vi "Write to TDMS(SubVI).vi"(8 "error in (no error)":errorcluster, 9 "LED state":string, 10 "element":T1 {"RMS" format="%0.6f"; "RPM" format="%0.2f"; "Voltage" format="%0.2f"; "Current" format="%0.2f"; "Temperature" format="%0.2f"}, 11 "Refnum in":refnum<k34>) -> (0 "error out":errorcluster, 3 "Refnum out":refnum<k34>)   [LabVIEW 2017]
uses:
  typedefs/Data.ctl
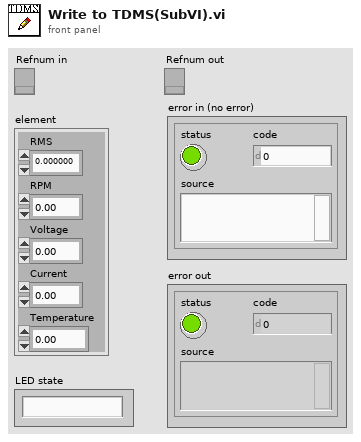
[diagram p1: front panel]
types:
  T1 = typedef "Data.ctl" = cluster{"RMS":dbl, "RPM":dbl, "Voltage":dbl, "Current":dbl, "Temperature":dbl}
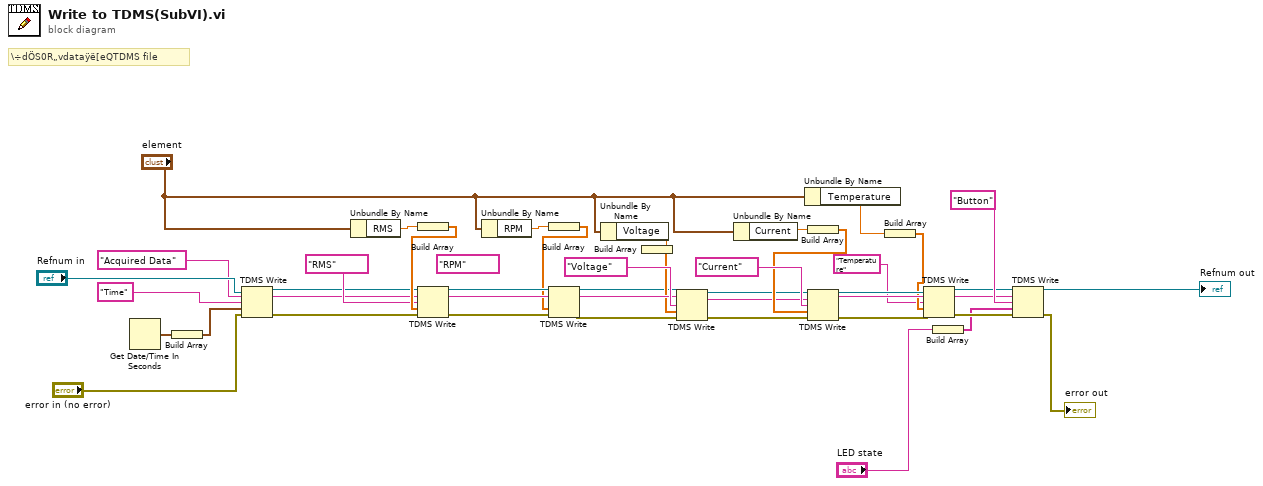
[diagram p0: block diagram]
diagram:
  (unwired) "RPM" ("group name in (Untitled)")
  # "\\÷dÖS0R„vdataÿë[eQTDMS file"
  n1 = Get Date/Time In Seconds() -> (seconds since 1Jan1904=w3:timestamp)
  n2 = Build Array(w3) -> (w4:timestamp[])
  n3 = TDMS Write(0:"Refnum in", 5:"Acquired Data" ("group name in (Untitled)"), 7:"Time" ("group name in (Untitled)"), 9:w4, 11:"error in (no error)") -> (4:w8:refnum<k34>, 6:w6:string, 15:w7:errorcluster)  [unwired: 1 in, 1 out]
  n4 = Unbundle By Name("element") -> ("RMS"=w9:dbl)
  n5 = Build Array(w9) -> (w11:dbl[])
  n6 = TDMS Write(0:w8, 5:w6, 7:"RMS" ("group name in (Untitled)"), 9:w11, 11:w7) -> (4:w14:refnum<k34>, 6:w15:string, 15:w16:errorcluster)  [unwired: 1 in, 1 out]
  n7 = Unbundle By Name("element") -> ("RPM"=w13:dbl)
  n8 = Build Array(w13) -> (w12:dbl[])
  n9 = TDMS Write(0:w14, 5:w15, 9:w12, 11:w16) -> (4:w22:refnum<k34>, 6:w25:string, 15:w24:errorcluster)  [unwired: 2 in, 1 out]
  n10 = Unbundle By Name("element") -> ("Voltage"=w21:dbl)
  n11 = Build Array(w21) -> (w23:dbl[])
  n12 = TDMS Write(0:w22, 5:w25, 7:"Voltage" ("group name in (Untitled)"), 9:w23, 11:w24) -> (4:w19:refnum<k34>, 6:w18:string, 15:w17:errorcluster)  [unwired: 1 in, 1 out]
  n13 = Unbundle By Name("element") -> ("Current"=w20:dbl)
  n14 = Unbundle By Name("element") -> ("Temperature"=w31:dbl)
  n15 = Build Array(w20) -> (w27:dbl[])
  n16 = TDMS Write(0:w19, 5:w18, 7:"Current" ("group name in (Untitled)"), 9:w27, 11:w17) -> (4:w32:refnum<k34>, 6:w34:string, 15:w33:errorcluster)  [unwired: 1 in, 1 out]
  n17 = Build Array(w31) -> (w30:dbl[])
  n18 = TDMS Write(0:w32, 5:w34, 7:"Temperature" ("group name in (Untitled)"), 9:w30, 11:w33) -> (4:w37:refnum<k34>, 6:w36:string, 15:w41:errorcluster)  [unwired: 1 in, 1 out]
  n19 = Build Array("LED state") -> (w39:string[])
  n20 = TDMS Write(0:w37, 5:w36, 7:"Button" ("channel name(s) in (Untitled)"), 9:w39, 11:w41) -> (4:→"Refnum out":refnum<k34>, 15:→"error out":errorcluster)  [unwired: 1 in, 2 out]
